vi "json_cache_delete.vi"(8 "error in (no error)":errorcluster, 11 "cache id":u64) -> (0 "error out":errorcluster, 1 "exists?":bool, 3 "elements":T1[](array[typedef]))   [LabVIEW 2017]
uses:
  json_element.ctl
  json_element_type.ctl
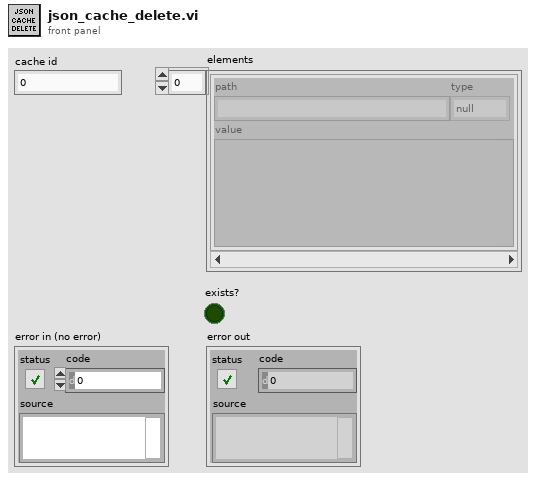
[diagram p1: front panel]
types:
  T1 = typedef "json_element.ctl" = cluster{"path":string, "type":T2, "value":variant}
  T2 = typedef "json_element_type.ctl" = enum8{"null", "bool", "int", "uint", "float", "string", "array", "object"}
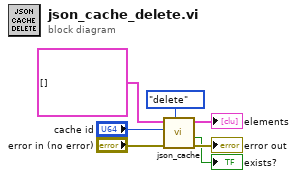
[diagram p0: block diagram]
diagram:
  n1 = call "json_cache.vi"("action"=enum8{"null", "get", "create", "delete"}."delete", "error in (no error)"="error in (no error)", "cache id in"="cache id", "elements in"=T1[] []) -> ("error out"=→"error out":errorcluster, "exists?"=→"exists?":bool, "elements out"=→"elements":T1[])  [unwired: 3 in, 2 out]
